vi "set_attenuation.vi"(8 "error in (no error)":errorcluster, 10 "Value":string, 11 "VISA Refnum in":refnum<visa-resource-name>) -> (0 "error out":errorcluster, 3 "VISA Refnum out":refnum<visa-resource-name>)   [LabVIEW 2015]
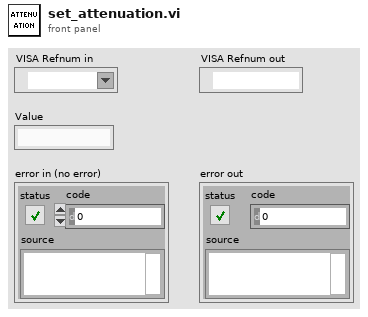
[diagram p1: front panel]
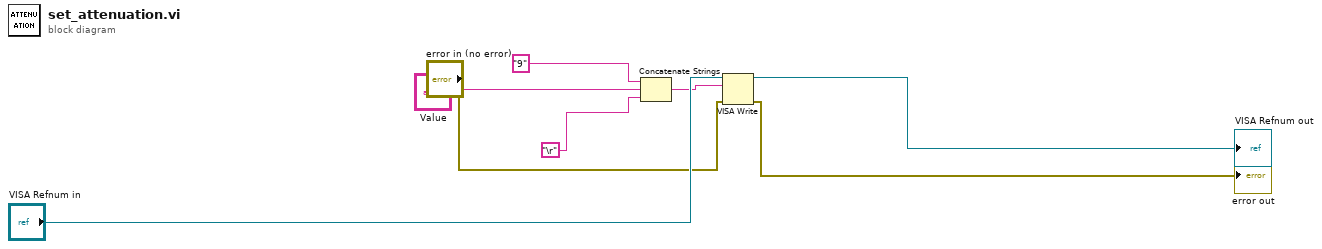
[diagram p0: block diagram]
diagram:
  n1 = Concatenate Strings("9" ("string"), "Value", "\r") -> (w2:string)
  n2 = VISA Write(VISA resource name="VISA Refnum in", write buffer=w2, error in (no error)="error in (no error)") -> (VISA resource name out=→"VISA Refnum out":refnum<visa-resource-name>, error out=→"error out":errorcluster)  [unwired: 1 out]
